vi "Open Excel sheet.vi"(6 "error in (no error)":errorcluster) -> (0 "error out":errorcluster, 1 "Excel._Application":refnum<k7>, 2 "Excel._Workbook":refnum<k7>, 3 "Excel._Worksheet":refnum<k7>)   [LabVIEW 2012]
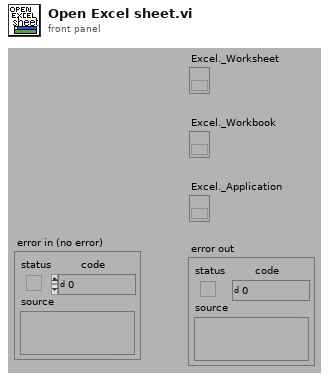
[diagram p1: front panel]
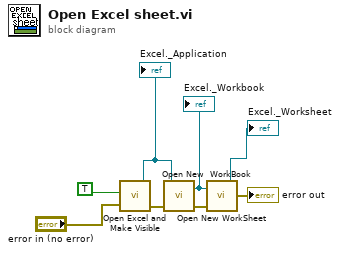
[diagram p0: block diagram]
diagram:
  n1 = call "Open Excel and Make Visible.vi"("error in (no error)"="error in (no error)", "Visible Boolean"=TRUE) -> ("error out"=w3:errorcluster, "Excel._Application"=w8:refnum<k7>)
  "Excel._Application" <- w8
  n2 = call "Open New  WorkBook.vi"("error in (no error)"=w3, "Excel._Application"=w8) -> ("error out"=w4:errorcluster, "Excel._Workbook"=w7:refnum<k7>)  [unwired: 1 in]
  "Excel._Workbook" <- w7
  n3 = call "Open New WorkSheet.vi"("error in (no error)"=w4, "Excel._Workbook"=w7) -> ("error out"=→"error out":errorcluster, "Excel._Worksheet"=→"Excel._Worksheet":refnum<k7>)  [unwired: 1 in]
